vi "daqhat_tcp_clock.vi"(8 "error in (no error)":errorcluster, 10 "Desired frequency":dbl, 11 "TCP network connection in":refnum<k5>) -> (0 "error out":errorcluster, 2 "Set frequency":dbl, 3 "TCP Network Connection out":refnum<k5>)   [LabVIEW 2018]
doc: "Set MCC 172 ADC sampling frequency using a TCP server running on a Raspberry Pi. The TCP server program must be running on the Pi, and the TCP connection already opened to the correct IP address and port. Provide the frequency in Hz. The actual frequency set will be returned."
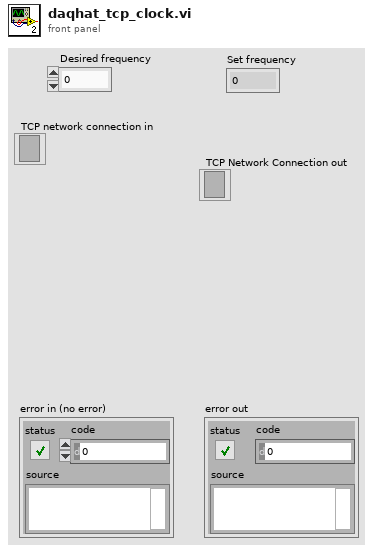
[diagram p1: front panel]
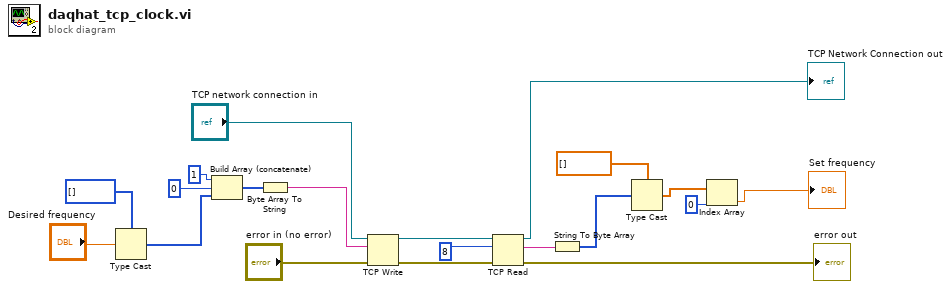
[diagram p0: block diagram]
diagram:
  n1 = Type Cast(type=u8[] [], x="Desired frequency") -> (*(type *) &x=w3:u8[])
  n2 = Build Array (concatenate)(u8 1, u8 0, w3) -> (w20:u8[])
  n3 = Byte Array To String(unsigned byte array=w20) -> (string=w5:string)
  n4 = TCP Write(connection ID="TCP network connection in", data in=w5, error in (no error)="error in (no error)") -> (connection ID out=w17:refnum<k5>, error out=w18:errorcluster)  [unwired: 1 in, 1 out]
  n5 = TCP Read(connection ID=w17, bytes to read=8, error in (no error)=w18) -> (connection ID out=→"TCP Network Connection out":refnum<k5>, data out=w1:string, error out=→"error out":errorcluster)  [unwired: 2 in]
  n6 = String To Byte Array(string=w1) -> (unsigned byte array=w9:u8[])
  n7 = Type Cast(type=dbl[] [], x=w9) -> (*(type *) &x=w8:dbl[])
  n8 = Index Array(array=w8, index=0) -> (element=→"Set frequency":dbl)
